vi "Fit Transform.vi"(7 "Type X":T1(ring), 8 "error in (no error)":errorcluster caption="entrée d'erreur (pas d'erreur)", 9 "y":string[][](array[string]), 10 "X":string[][](array[string]), 11 "SimpleImputer.lvclass":refnum<class "SimpleImputer.lvclass">) -> (0 "error out":errorcluster caption="sortie d'erreur", 2 "Data":T2, 3 "SimpleImputer.lvclass":refnum<class "SimpleImputer.lvclass">)   [LabVIEW 2020, in "SimpleImputer.lvclass"]
doc: "Fit to data, then transform it.\n\nFits transformer to X and y with optional parameters fit_params and returns a transformed version of X.\n\nReturns : \n\n- X_new : ndarray array of shape (n_samples, n_features_new)\nTransformed array."
uses:
  SimpleImputer.lvclass
  SimpleImputer.lvclass/SimpleImputer.ctl
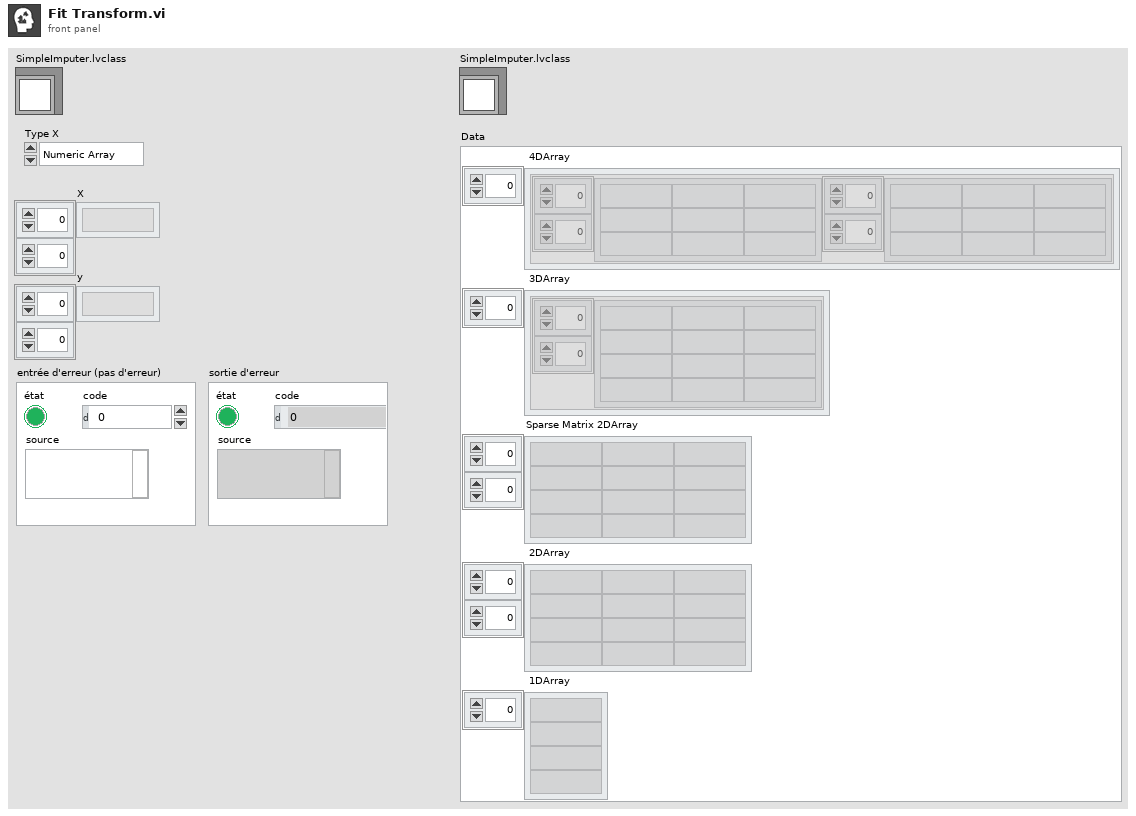
[diagram p1: front panel]
types:
  T1 = enum16{"Numeric Array", "String Array", "Sparse"}
  T2 = cluster{" 4DArray":cluster{"1":string[][], "2":string[][]}[], " 3DArray":cluster{"Tableau":string[][]}[], "Sparse Matrix 2DArray":string[][], " 2DArray":string[][], " 1DArray":string[]}
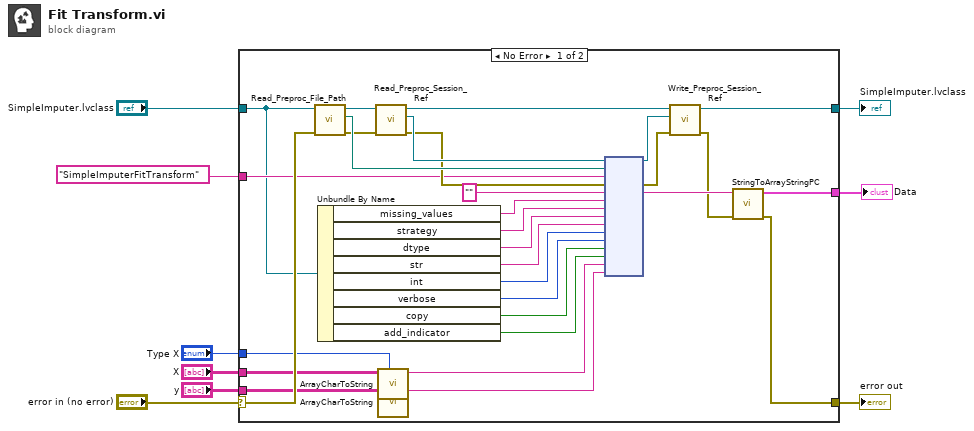
[diagram p0: block diagram]
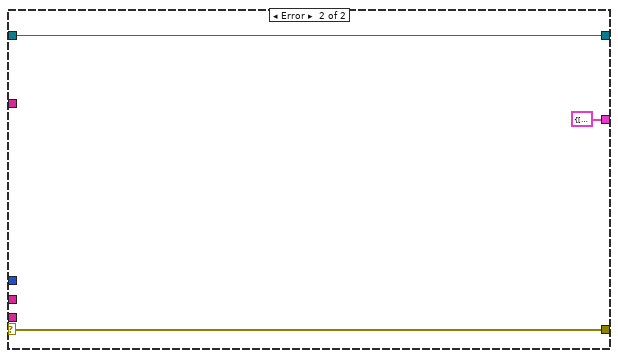
[diagram p2: hidden frame]
diagram:
  n1 = case shown="No Error" "error in (no error)" {
    selector: "error in (no error)" -> [w30 w42]
    tunnel: [w16 w42] -> w8
    tunnel: [w19 w41] -> w6
    tunnel: "SimpleImputer.lvclass" -> [w28 w41]
    tunnel: "SimpleImputerFitTransform" ("Fonction") -> [w29 _]
    tunnel: "X" -> [w14 _]
    tunnel: "y" -> [w11 _]
    tunnel: "Type X" -> [w12 _]
    tunnel: [w15 T2 {" 4DArray"=[], " 3DArray"=[], "Sparse Matrix 2DArray"=[], " 2DArray"=[], " 1DArray"=[]} ("Data")] -> w1
    frame No Error {
      n2 = call-dynamic "Read_Preproc_File_Path.vi"("error in (no error)"=w30, "Python in"=w28) -> ("error out"=w34:errorcluster, "File_Path"=w37:path, "Python out"=w39:refnum<class "SimpleImputer.lvclass">)  [unwired: 7 in]
      n3 = Unbundle By Name(w28) -> ("missing_values"=w27:string, "strategy"=w26:string, "dtype"=w25:string, "str"=w24:string, "int"=w23:i32, "verbose"=w22:i32, "copy"=w21:bool, "add_indicator"=w20:bool)
      n4 = call-dynamic "Read_Preproc_Session_Ref.vi"("error in (no error)"=w34, "Python in"=w39) -> ("error out"=w35:errorcluster, "Session_ref"=w36:refnum<k35>, "Python out"=w38:refnum<class "SimpleImputer.lvclass">)  [unwired: 7 in]
      n5 = call "ArrayCharToString.vi"("Type"=w12, "TAB"=w14) -> ("Instruction"=w13:string)  [unwired: 9 in]
      n6 = call "ArrayCharToString.vi"("TAB"=w11) -> ("Instruction"=w10:string)  [unwired: 10 in]
      n7 = node(w36, w37, w29, w35, "", w27, w26, w25, w24, w23, w22, w21, w20, w13, w10) -> (w31:refnum<k35>, w33:errorcluster, w18:string)  [unwired: 10 in, 2 out]
      n8 = call-dynamic "Write_Preproc_Session_Ref.vi"("error in (no error)"=w33, "Session_ref"=w31, "Python in"=w38) -> ("error out"=w17:errorcluster, "Python out"=w19:refnum<class "SimpleImputer.lvclass">)  [unwired: 7 in]
      n9 = call "StringToArrayStringPC.vi"("sortie d'erreur"=w17, "Return value"=w18) -> ("sortie d'erreur"=w16:errorcluster, "Data"=w15:T2)  [unwired: 8 in]
    }
    frame Error {
    }
  }
  "error out" <- w8
  "SimpleImputer.lvclass" <- w6
  "Data" <- w1
